vi "表格自动移位.vi"(8 "错误输入（无错误）":errorcluster, 9 "一页行数":u32, 11 "表格引用输入":refnum<vi>) -> (0 "错误输出":errorcluster, 3 "引用输出":refnum<vi>)   [LabVIEW 2014, in "表格.lvlib"]
uses:
  <vilib>/Utility/miscctls.llb/LVRowAndColumnUnsignedTypeDef.ctl
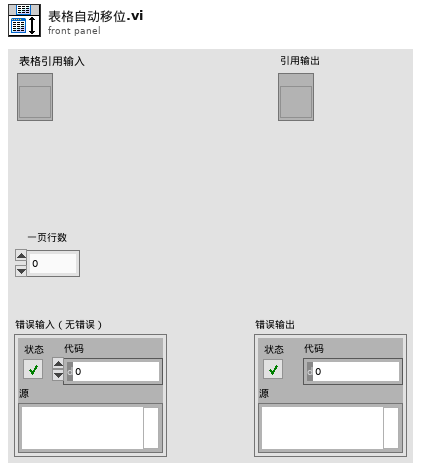
[diagram p1: front panel]
types:
  T1 = typedef "LVRowAndColumnUnsignedTypeDef.ctl" = cluster{"Row":u32, "Column":u32}
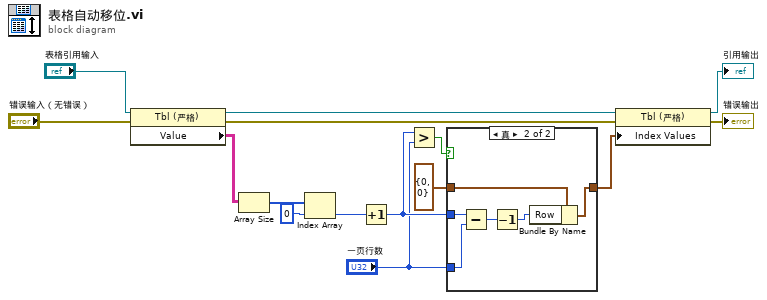
[diagram p0: block diagram]
diagram:
  n1 = property class="Tbl (严格)"(reference="表格引用输入", error in="错误输入（无错误）") -> (reference out=w7:refnum<vi>, error out=w2:errorcluster, "Value"=w6:string[][])
  n2 = Array Size(array=w6) -> (size(s)=w5:i32[])
  n3 = Index Array(array=w5, index=0 ("索引")) -> (element=w3:i32)
  n4 = Increment(x=w3) -> (x+1=w13:i32)
  n5 = Greater?(x=w13, y="一页行数") -> (0:w14:bool)
  n6 = case shown="真" w14 {
    tunnel: T1 {"Row"=0, "Column"=0} ("索引值") -> [w16 w22]
    tunnel: [w16 w21] -> w12
    tunnel: w13 -> [_ w19]
    tunnel: "一页行数" -> [_ w18]
    frame False {
    }
    frame True {
      n7 = Subtract(x=w19, y=w18) -> (x-y=w20:u32)
      n8 = Decrement(x=w20) -> (x-1=w17:u32)
      n9 = Bundle By Name(cluster=w22, "Row"=w17) -> (w21:T1)
    }
  }
  n10 = property class="Tbl (严格)"(reference=w7, error in=w2, "Index Values"=w12) -> (reference out=→"引用输出":refnum<vi>, error out=→"错误输出":errorcluster)
